vi "Detect Rising Edge.vi"(10 "signal":bool) -> (2 "edge detected":bool)   [LabVIEW 2018]
doc: "Generates TRUE once <b>signal</b> changes from false to true."
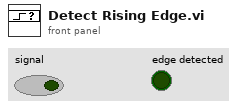
[diagram p1: front panel]
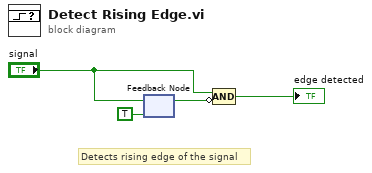
[diagram p0: block diagram]
diagram:
  # "Detects rising edge of the signal"
  n1 = feedback #1(TRUE) -> (w3:bool)
  n2 = feedback-in #1("signal") -> ()
  n3 = Compound Arithmetic op=AND("signal", invert w3) -> (→"edge detected":bool)
